vi "Release Public Key.vi"(8 "error in (no error)":errorcluster, 11 "public key":T1) -> (0 "error out":errorcluster)   [LabVIEW 2013, in "libssh2.lvlib"]
doc: "Releases all resources associated with <B>public key</B>."
uses:
  libssh2.lvlib
  Public Key Refnum.ctl
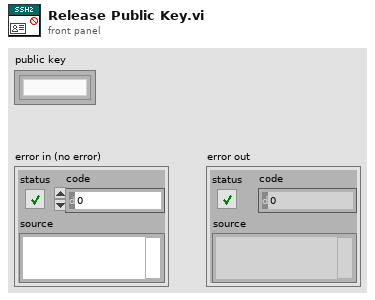
[diagram p1: front panel]
types:
  T1 = typedef "libssh2.lvlib/Public Key Refnum.ctl" = refnum<k1>
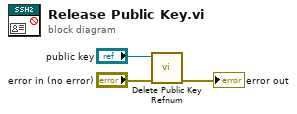
[diagram p0: block diagram]
diagram:
  n1 = call "Delete Public Key Refnum.vi"("error in (no error)"="error in (no error)", "public key"="public key") -> ("error out"=→"error out":errorcluster)  [unwired: 8 in, 1 out]
